vi "Handle Error (User).vi"(8 "error in":errorcluster, 11 "Node in":refnum<class "AMS Power Supply Template.lvclass">) -> (0 "error out":errorcluster, 3 "Node out":refnum<class "AMS Power Supply Template.lvclass">)   [LabVIEW 2023, in "AMS Power Supply Template.lvlib" / "AMS Power Supply Template.lvclass"]
uses:
  AMS Power Supply Template.lvclass
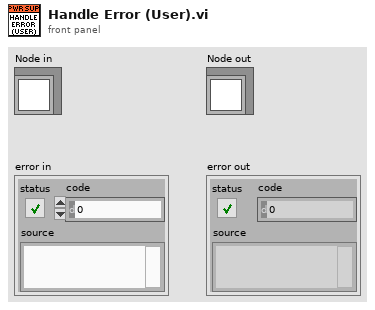
[diagram p1: front panel]
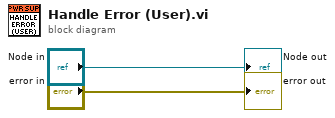
[diagram p0: block diagram]
diagram:
  "error out" <- "error in"
  "Node out" <- "Node in"
